vi "Image Queue.vi"(7 "Action":T2=enum."Enqueue", 8 "Error In":errorcluster, 11 "Image In":T1) -> (0 "Error Out":errorcluster, 3 "Image Out":T1)   [LabVIEW 2018]
uses:
  Controls/Queue Manager Actions.ctl
  <vilib>/vision/Image Controls.llb/IMAQ Image.ctl
  Controls/MessagePacket.ctl
  Controls/QueueNames.ctl
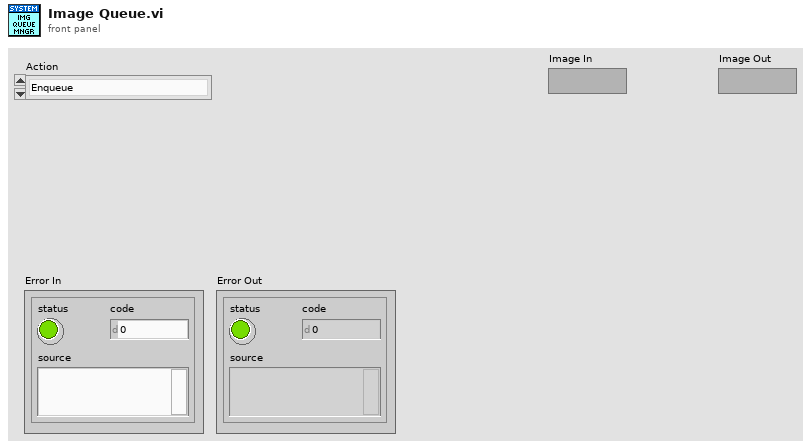
[diagram p1: front panel]
types:
  T1 = typedef "IMAQ Image.ctl" = refnum<image>
  T2 = typedef "Queue Manager Actions.ctl" = enum16{"Init", "Enqueue", "Enqueue All", "Preview Queue", "Dequeue", "Get Status", "Flush Queue", "Flush All Queues", "Release All Queues", "Release Queue", "Enqueue at Opposite End"}
  T3 = typedef "MessagePacket.ctl" = cluster{"Message":string, "Parameter":variant}
  T4 = typedef "QueueNames.ctl" = enum16{"Main GUI", "Main Scan Processor", "Main Processing", "Main Saving", "Main Display", "Main Table Stage GUI", "Main Table Stage Proc.", "Scan Engine", "Vibratome GUI", "Vibratome Processor", "Slice Engine"}
  T5 = typedef "Image Type" = u32
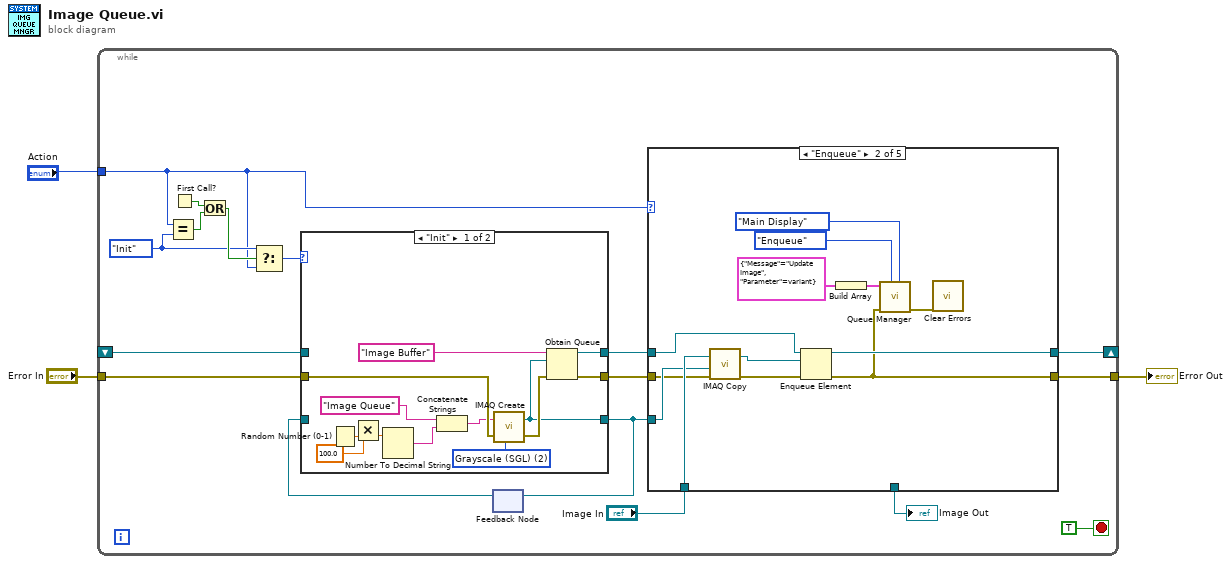
[diagram p0: block diagram]
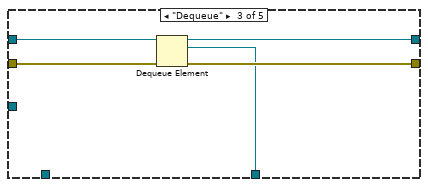
[diagram p3: hidden frame]
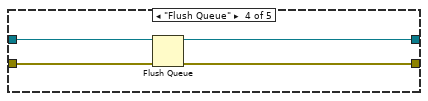
[diagram p4: hidden frame]
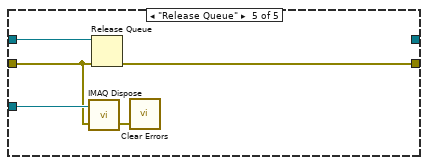
[diagram p5: hidden frame]
diagram:
  n1 = while {
    tunnel: "Action" -> [w8]
    tunnel: "Error In" -> [w15]
    tunnel: [w14] -> w1
    shift-right: [w10] -> _
    shift-left: _ -> [w9]
    stop <- TRUE stop-if-true
    w17 = Queue_Manager_Actions."Init"
    n2 = Equal?(x=w8, y=w17) -> (x = y?=w19:bool)
    n3 = First Call?() -> (First Call?: T/F=w20:bool)
    n4 = Or(x=w20, y=w19) -> (x .or. y?=w18:bool)
    n5 = Select(t=w17, s=w18, f=w8) -> (s? t:f=w16:T2)
    n6 = feedback #1() -> (w5:T1)  [unwired: 1 in]
    n7 = case shown="\"Init\"" w16 {
      tunnel: [w62 w64] -> w12
      tunnel: w15 -> [w57 w65]
      tunnel: [w61 w65] -> w13
      tunnel: w9 -> [_ w64]
      tunnel: [w56 w63] -> w6
      tunnel: w5 -> [_ w63]
      frame "Init" {
        w50 = T5 2 items=["Grayscale (U8)", "Grayscale (I16)", "Grayscale (SGL)", "Complex (CSG)", "RGB (U32)", "HSL (U32)", "RGB (U64)", "Grayscale (U16)"] ("Image Type")
        n8 = Random Number (0-1)() -> (number: 0 to 1=w52:dbl)
        n9 = Multiply(x=100.0, y=w52) -> (x*y=w53:dbl)
        n10 = Number To Decimal String(number=w53) -> (decimal integer string=w51:string)  [unwired: 1 in]
        n11 = Concatenate Strings("Image Queue" ("Image Name"), w51) -> (w55:string)
        n12 = call "IMAQ Create"("Image Name"=w55, "Image Type"=w50, "error in (no error)"=w57) -> ("New Image"=w56:T1, "error out"=w58:errorcluster)  [unwired: 2 in]
        n13 = Obtain Queue(name (unnamed)="Image Buffer", element data type=w56, error in (no error)=w58) -> (queue out=w62:refnum<queue>, error out=w61:errorcluster)  [unwired: 2 in, 1 out]
      }
      frame "Enqueue", Default {
      }
    }
    n14 = feedback-in #1(w6) -> ()
    n15 = case shown="\"Enqueue\"" w8 {
      tunnel: w12 -> [w21 w31 w37 w42 w48]
      tunnel: [w22 w24 w39 w43 w49] -> w14
      tunnel: w13 -> [w22 w33 w40 w44 w46]
      tunnel: [_ _ w38 _ _] -> w7
      tunnel: [w21 w29 w36 w41 _] -> w10
      tunnel: w6 -> [_ w34 _ _ w47]
      tunnel: "Image In" -> [_ w35 _ _ _]
      frame "Init", Default {
      }
      frame "Enqueue" {
        n16 = call "IMAQ Copy"("error in (no error)"=w33, "Image Dst"=w34, "Image Src"=w35) -> ("error out"=w32:errorcluster, "Image Dst Out"=w30:T1)  [unwired: 3 in]
        n17 = Enqueue Element(queue=w31, element=w30, error in (no error)=w32) -> (queue out=w29:refnum<queue>, error out=w24:errorcluster)  [unwired: 1 in, 1 out]
        n18 = Build Array(T3 {"Message"="Update Image", "Parameter"=variant} ("Message Packet [In]")) -> (w25:T3[])
        n19 = call "Queue Manager.vi"("Queue Name"=QueueNames."Main Display", "Action"=Queue_Manager_Actions."Enqueue", "Error In"=w24, "Message Packet Array"=w25) -> ("Error Out"=w23:errorcluster)  [unwired: 3 in, 4 out]
        n20 = call <vilib>:"Clear Errors.vi"("error in (no error)"=w23) -> ()  [unwired: 5 in, 2 out]
      }
      frame "Dequeue" {
        n21 = Dequeue Element(queue=w37, error in (no error)=w40) -> (queue out=w36:refnum<queue>, element=w38:T1, error out=w39:errorcluster)  [unwired: 1 in, 1 out]
      }
      frame "Flush Queue" {
        n22 = Flush Queue(queue=w42, error in (no error)=w44) -> (queue out=w41:refnum<queue>, error out=w43:errorcluster)  [unwired: 1 out]
      }
      frame "Release Queue" {
        n23 = call "IMAQ Dispose"("Image"=w47, "error in (no error)"=w46) -> ("error out"=w45:errorcluster)  [unwired: 4 in]
        n24 = Release Queue(queue=w48, error in (no error)=w46) -> (error out=w49:errorcluster)  [unwired: 1 in, 2 out]
        n25 = call <vilib>:"Clear Errors.vi"("error in (no error)"=w45) -> ()  [unwired: 5 in, 2 out]
      }
    }
    "Image Out" <- w7
  }
  "Error Out" <- w1
